vi "Attempt-create-client.vi"(8 "error in (no error)":errorcluster, 9 "Module path":path, 10 "Module type":string, 11 "ModComm in":T1) -> (0 "error out":errorcluster, 3 "ModComm out":T1)   [LabVIEW 2013, in "SLMServer.lvlib" / "SLMServer.lvclass"]
uses:
  SLMServer.lvclass
  Object-reference.ctl
  UI-messages.ctl
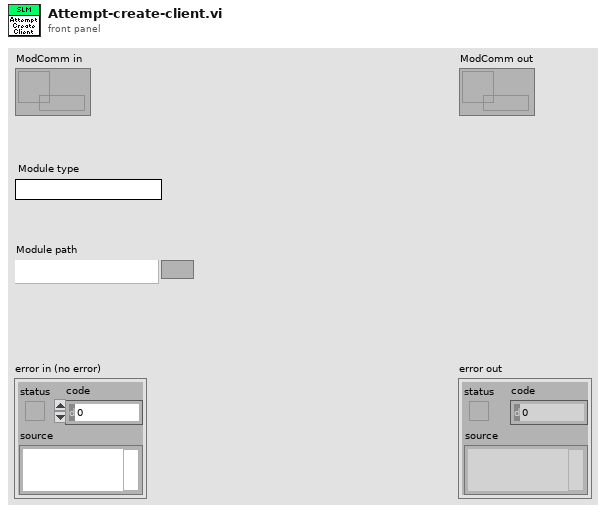
[diagram p1: front panel]
types:
  T1 = typedef "SLMServer.lvlib/SLMServer.lvclass/Object-reference.ctl" = refnum<data-value>
  T2 = typedef "SLMServer.lvlib/SLMServer.lvclass/UI-messages.ctl" = enum16{"Time out", "User cancel", "Module cancel", "Client inactivity", "Client limit", "Client started"}
  T3 = typedef "SLMServer.lvlib/SLMServer.lvclass/Supported-module-types.ctl" = enum16{"SLMControl", "PowderDeposition", "CameraVision", "Server", "All", "StrategyParser", "MaterialCharacterization", "StatusMonitor", "SLMSimulation", "LaserCharacterization"}
  T4 = enum32{"invalid app kind", "Development System", "Run Time System", "Student Edition", "Embedded LabVIEW", "Evaluation", "Custom"}
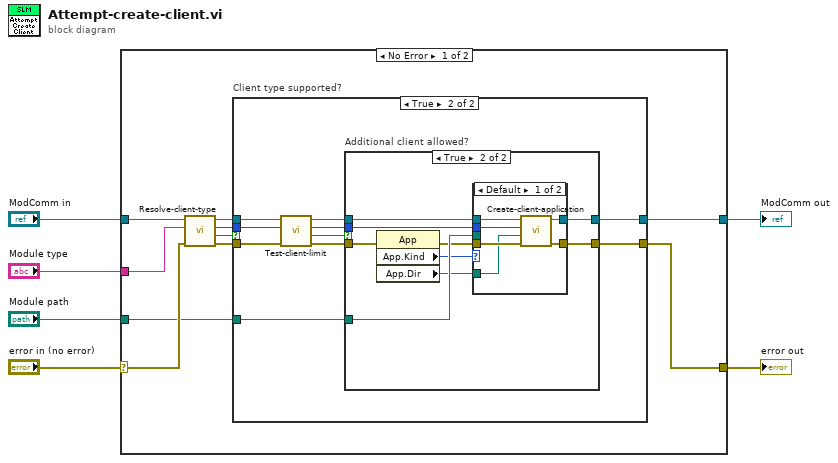
[diagram p0: block diagram]
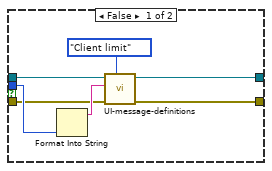
[diagram p3: hidden frame]
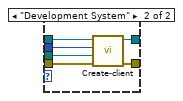
[diagram p4: hidden frame]
diagram:
  n1 = case shown="No Error" "error in (no error)" {
    selector: "error in (no error)" -> [w10 w58]
    tunnel: [w8 w58] -> w5
    tunnel: [w9 w57] -> w3
    tunnel: "ModComm in" -> [w16 w57]
    tunnel: "Module type" -> [w15 _]
    tunnel: "Module path" -> [w7 _]
    frame No Error {
      n2 = call "Resolve-client-type.vi"("error in (no error)"=w10, "Module name"=w15, "ModComm in"=w16) -> ("error out"=w11:errorcluster, "Supported?"=w13:bool, "Module type"=w12:T3, "ModComm out"=w14:T1)  [unwired: 5 in]
      n3 = case "Client type supported?" shown="True" w13 {
        tunnel: w14 -> [w18 w28]
        tunnel: w12 -> [_ w26]
        tunnel: w11 -> [w17 w27]
        tunnel: [w18 w21] -> w9
        tunnel: [w17 w20] -> w8
        tunnel: w7 -> [_ w19]
        frame False {
        }
        frame True {
          n4 = call "Test-client-limit.vi"("error in (no error)"=w27, "Module type"=w26, "ModComm in"=w28) -> ("error out"=w24:errorcluster, "Client allowed?"=w25:bool, "Module type dup"=w22:T3, "ModComm out"=w23:T1)  [unwired: 5 in]
          n5 = case "Additional client allowed?" shown="True" w25 {
            tunnel: w24 -> [w31 w39]
            tunnel: w23 -> [w32 w44]
            tunnel: w22 -> [w33 w41]
            tunnel: [w29 w43] -> w21
            tunnel: [w30 w42] -> w20
            tunnel: w19 -> [_ w40]
            frame False {
              n6 = Format Into String(w33) -> (resulting string=w34:string)  [unwired: 3 in, 1 out]
              n7 = call "UI-message-definitions.vi"("Message"=UI-messages."Client limit", "error in (no error)"=w31, "Additional text"=w34, "ModComm in"=w32) -> ("error out"=w30:errorcluster, "ModComm out"=w29:T1)  [unwired: 6 in]
            }
            frame True {
              n8 = property class="App"(error in=w39) -> (error out=w38:errorcluster, "App.Kind"=w37:T4, "App.Dir"=w36:path)  [unwired: 1 in, 1 out]
              n9 = case shown="Default" w37 {
                tunnel: w44 -> [w50 w56]
                tunnel: [w48 w55] -> w43
                tunnel: [w47 w54] -> w42
                tunnel: w41 -> [w46 w53]
                tunnel: w40 -> [_ w52]
                tunnel: w38 -> [w49 w51]
                tunnel: w36 -> [w45 _]
                frame Default {
                  n10 = call "Create-client-application.vi"("error in (no error)"=w49, "Module path"=w45, "Module type"=w46, "ModComm in"=w50) -> ("error out"=w47:errorcluster, "ModComm out"=w48:T1)  [unwired: 6 in]
                }
                frame "Development System" {
                  n11 = call "Create-client.vi"("error in (no error)"=w51, "Module path"=w52, "Module type"=w53, "ModComm in"=w56) -> ("error out"=w54:errorcluster, "ModComm out"=w55:T1)  [unwired: 6 in]
                }
              }
            }
          }
        }
      }
    }
    frame Error {
    }
  }
  "error out" <- w5
  "ModComm out" <- w3
